vi "Excel_Add_Waveform.vi"(7 "orientation (1d only)":enum16{"Vertical", "Horizontal"}(ring), 8 "error In":errorcluster, 9 "Waweform":waveform(dbl)[](array[waveform]), 10 "Excel start location":string, 11 "Ref In":T1) -> (0 "error out":errorcluster, 3 "duplicate reference":T1)   [LabVIEW 2013]
uses:
  excel.llb/excel Object Reference.ctl
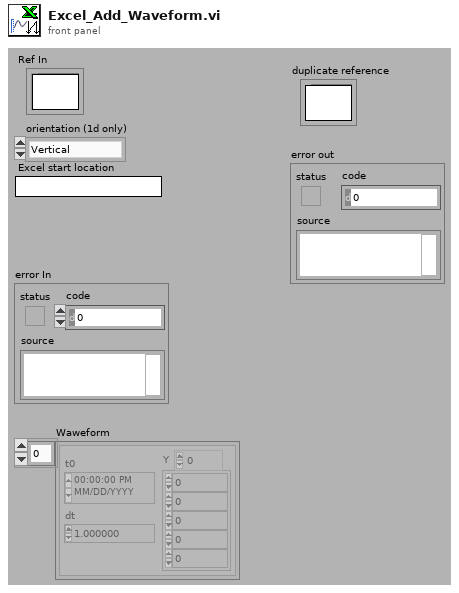
[diagram p1: front panel]
types:
  T1 = typedef "excel Object Reference.ctl" = refnum<k1>
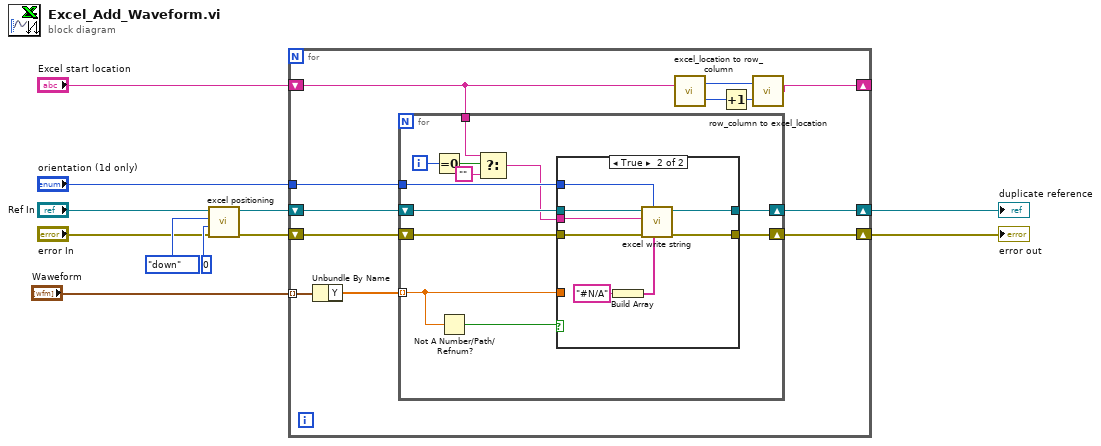
[diagram p0: block diagram]
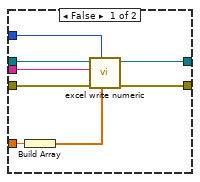
[diagram p2: hidden frame]
diagram:
  n1 = call "excel positioning.vi"("error in (no error)"="error In", "gap(0)"=0 ("gap"), "direction (right)"=enum16{"right", "down"}."down" ("direction"), "reference"="Ref In") -> ("error out"=w1:errorcluster, "duplicate reference"=w2:T1)  [unwired: 6 out]
  n2 = for {
    shift-right: [w13] -> w8
    shift-left: w2 -> [w18]
    shift-right: [w12] -> w7
    shift-left: w1 -> [w17]
    tunnel: "Waweform" -> [w23] mode=indexing
    tunnel: "orientation (1d only)" -> [w16]
    shift-right: [w22] -> _
    shift-left: "Excel start location" -> [w14]
    n3 = Unbundle By Name(w23) -> ("Y"=w15:dbl[])
    n4 = for {
      tunnel: w16 -> [w31]
      tunnel: w15 -> [w32] mode=indexing
      shift-right: [w24] -> w13
      shift-left: w18 -> [w34]
      shift-right: [w25] -> w12
      shift-left: w17 -> [w33]
      tunnel: w14 -> [w27]
      i -> [w30]
      n5 = Equal To 0?(x=w30) -> (x = 0?=w29:bool)
      n6 = Not A Number/Path/Refnum?(number/path/refnum=w32) -> (NaN/Path/Refnum?=w35:bool)
      n7 = Select(t=w27, s=w29, f="") -> (s? t:f=w26:string)
      n8 = case shown="True" w35 {
        tunnel: w34 -> [w43 w51]
        tunnel: w33 -> [w42 w50]
        tunnel: w32 -> [w41 _]
        tunnel: w31 -> [w39 w46]
        tunnel: w26 -> [w38 w47]
        tunnel: [w37 w48] -> w25
        tunnel: [w36 w49] -> w24
        frame False {
          n9 = Build Array(w41) -> (w40:dbl[])
          n10 = call "excel write numeric.vi"("Array 1d"=w40, "orientation (1d only)"=w39, "error in (no error)"=w42, "Excel_location"=w38, "reference"=w43) -> ("error out"=w37:errorcluster, "duplicate reference"=w36:T1)  [unwired: 1 in, 4 out]
        }
        frame True {
          n11 = Build Array("#N/A") -> (w44:string[])
          n12 = call "excel write string.vi"("1dArray"=w44, "orientation (1d only)"=w46, "error in (no error)"=w50, "Excel_location"=w47, "reference"=w51) -> ("error out"=w48:errorcluster, "duplicate reference"=w49:T1)  [unwired: 1 in, 4 out]
        }
      }
    }
    n13 = call "excel_location to row_column.vi"("Excel_location"=w14) -> ("Row"=w21:i32, "Column"=w20:i32)
    n14 = Increment(x=w20) -> (x+1=w19:i32)
    n15 = call "row_column to excel_location.vi"("Column"=w19, "Row"=w21) -> ("Excel_location"=w22:string)
  }
  "duplicate reference" <- w8
  "error out" <- w7
